vi "Populate Tree from S3 bucket Example.vi"() -> ()   [LabVIEW 2020]
uses:
  <vilib>/AWS Toolkit/S3/Object Content.ctl
  <vilib>/AWS Toolkit/S3/Storage Class.ctl
  <vilib>/AWS Toolkit/S3/Owner.ctl
  Data.S3/Data.S3.lvclass
  <vilib>/AWS Toolkit/S3/NI_AWS_S3.lvlib
panel:
  in  "Tree":string(tree)
  in  "Bucket name":string="levylab-data"
  in  "path to aws credentials":path
  out "Common Prefixes":string[](array[string])
  out "Objects in bucket":T1[](array[typedef])
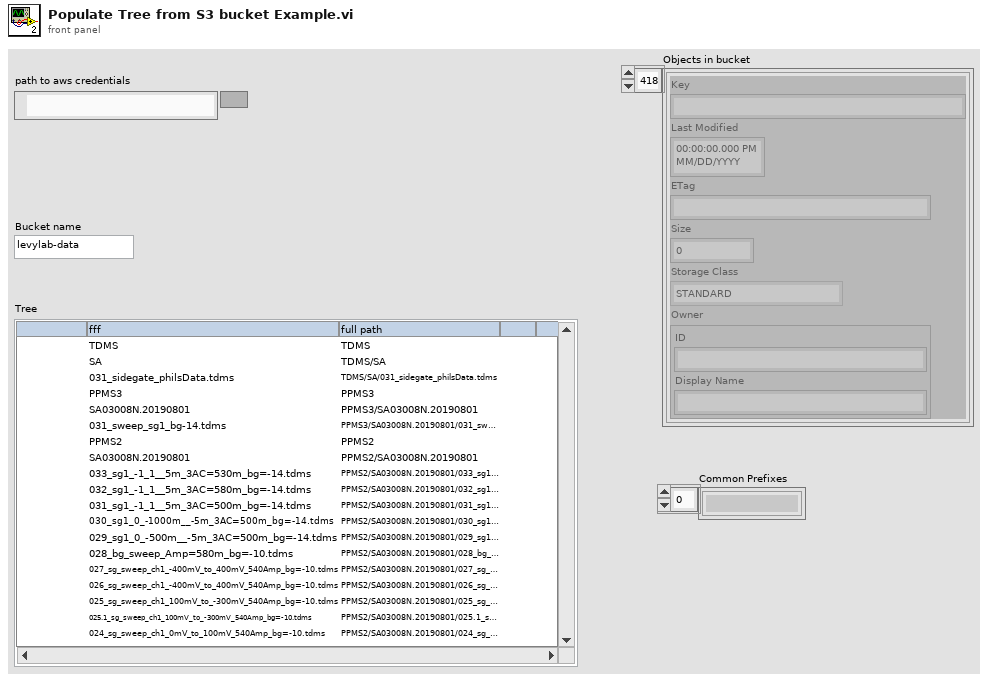
[diagram p1: front panel]
types:
  T1 = typedef "NI_AWS_S3.lvlib/Object Content.ctl" = cluster{"Key":string, "Last Modified":timestamp, "ETag":string, "Size":u64, "Storage Class":T2, "Owner":T3}
  T2 = typedef "NI_AWS_S3.lvlib/Storage Class.ctl" = enum16{"STANDARD", "REDUCED_REDUNDANCY"}
  T3 = typedef "NI_AWS_S3.lvlib/Owner.ctl" = cluster{"ID":string, "Display Name":string}
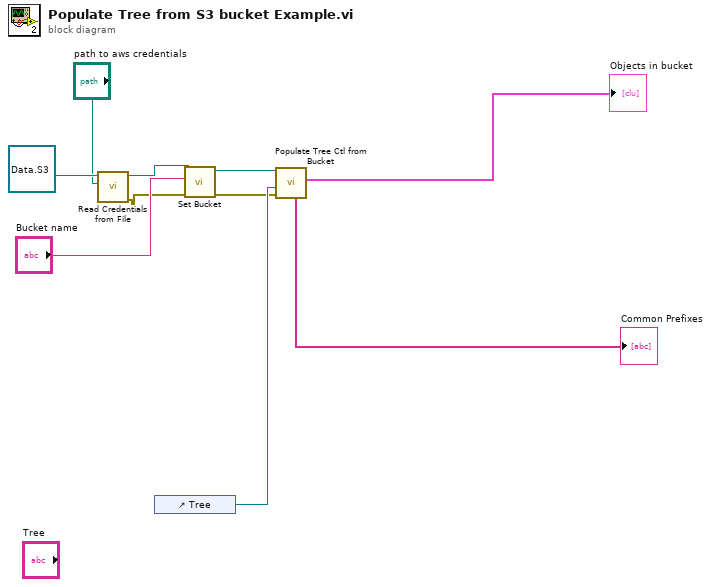
[diagram p0: block diagram]
diagram:
  n1 = call "Read Credentials from File.vi"("path to aws credentials"="path to aws credentials", "Data.S3"=refnum<class "Data.S3.lvclass"> refnum) -> ("error out"=w2:errorcluster, "Data.S3 out"=w6:refnum<class "Data.S3.lvclass">)  [unwired: 8 in]
  n2 = control-ref of="Tree"() -> (w10:refnum<vi>)
  n3 = call "Set Bucket.vi"("error in (no error)"=w2, "Bucket name"="Bucket name", "Data.S3 2"=w6) -> ("error out"=w1:errorcluster, "Data.S3"=w7:refnum<class "Data.S3.lvclass">)  [unwired: 7 in]
  n4 = call "Populate Tree Ctl from Bucket.vi"("error in (no error)"=w1, "Tree Ctl Ref"=w10, "Data.S3"=w7) -> ("Objects in bucket"=→"Objects in bucket":T1[], "Common Prefixes"=→"Common Prefixes":string[])  [unwired: 4 in, 3 out]
